vi "Auto Pickup Global.vi"() -> ()   [LabVIEW 2014]
panel:
  in  "Enable Auto Pickup":bool
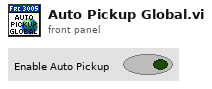
[diagram p1: front panel]
diagram:
